vi "ATF - DD Datalog and Display.vi"() -> ()   [LabVIEW 2022 SP3]
doc: "Datalog and display software modified"
uses:
  Source Code/Control/SeCrTs-Enum.ctl
  Source Code/Globals/SeCrTS-DD globals.vi
panel:
  in  "Control PC IP Address":string="169.254.57.227"
  out "Backlog Storage":i32
  out "Backlog Pump":i32
  out "Logging Mode":string
  out "cmd":bool=TRUE
  out "Storage Connected?":bool
  in  "Pump IP Address":string="169.254.31.109"
  in  "Storage IP Address":string="169.254.219.4"
  out "Datalog Title":string
  in  "Exit":bool
  out "Log Period(Min)":dbl
  out "Logging?":bool
  out "Pumb Connected?":bool
  out "error Out":errorcluster
  # "ATF PUMP AND STORAGE"
  # "DATALOG AND DISPLAY SOFTWARE"
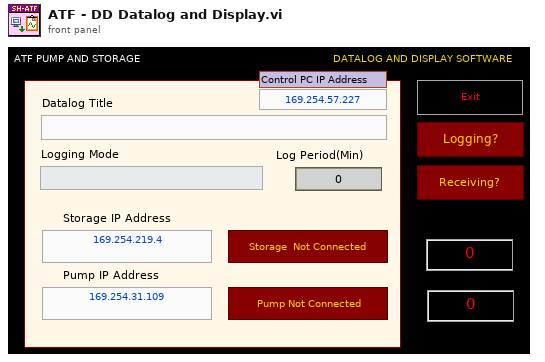
[diagram p1: front panel]
types:
  T1 = typedef "SeCrTs-Enum.ctl" = enum16{"Initialize", "Poll", "Establish ref", "Read", "Close", "Exit"}
  T2 = typedef "SeCrTS-Notifier Ref.ctl" = cluster{"Pump":refnum<notifier>, "Storage":refnum<notifier>}
  T3 = enum8{"Enabled", "Disabled", "Disabled and Grayed Out"}
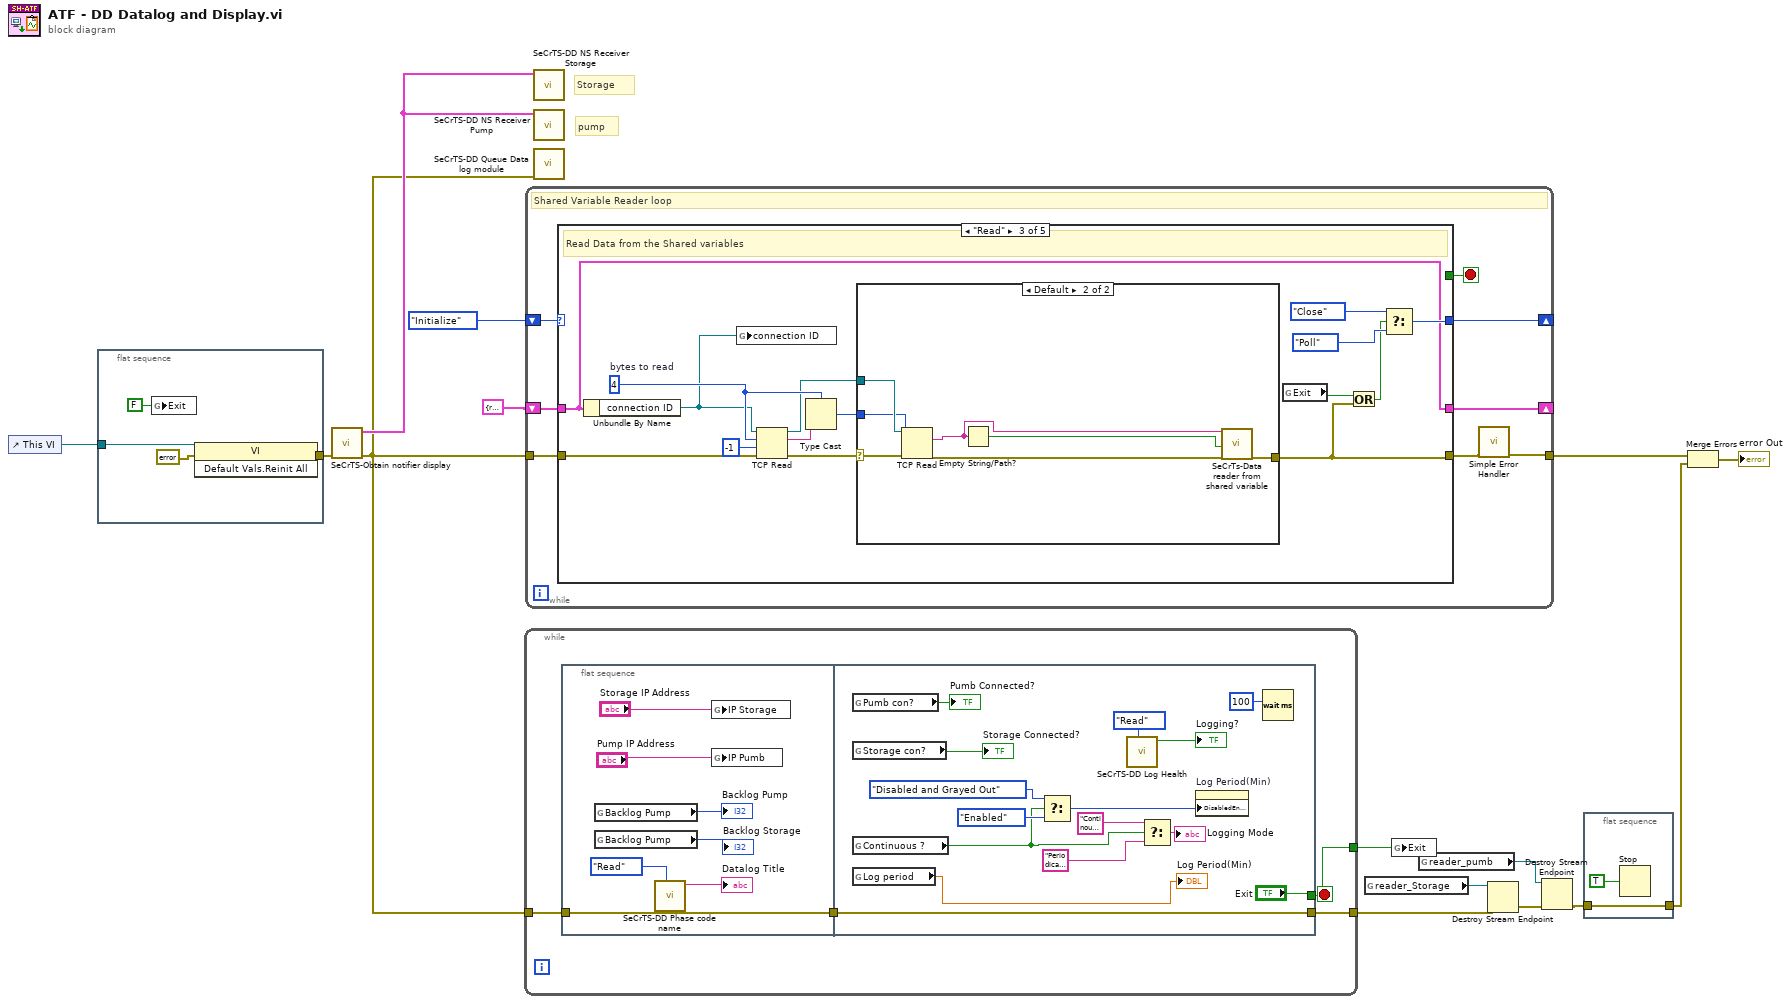
[diagram p0: block diagram]
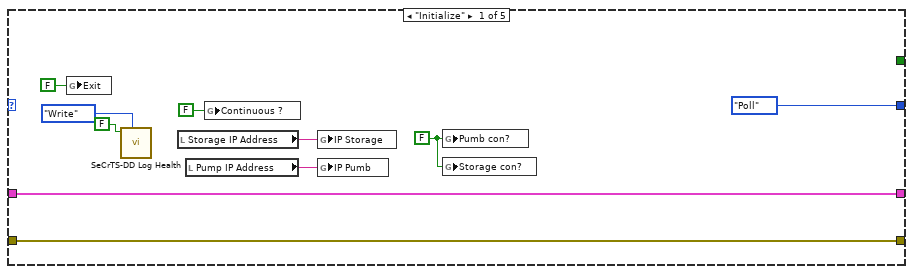
[diagram p2: hidden frame]
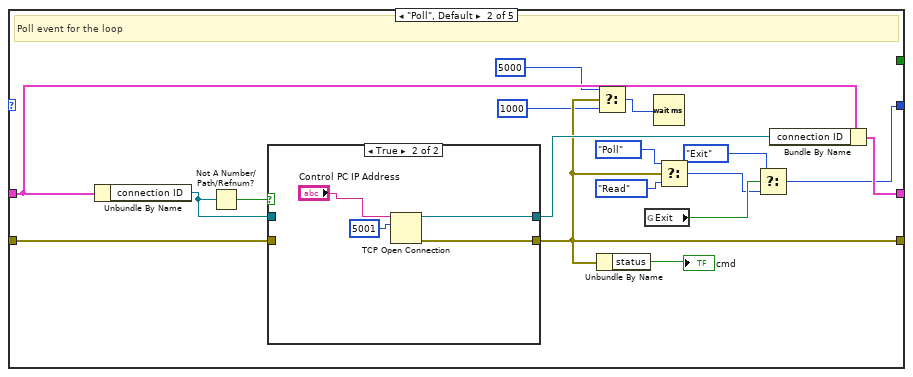
[diagram p3: hidden frame]
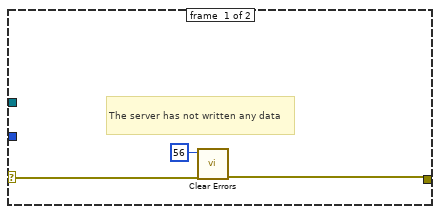
[diagram p5: hidden frame]
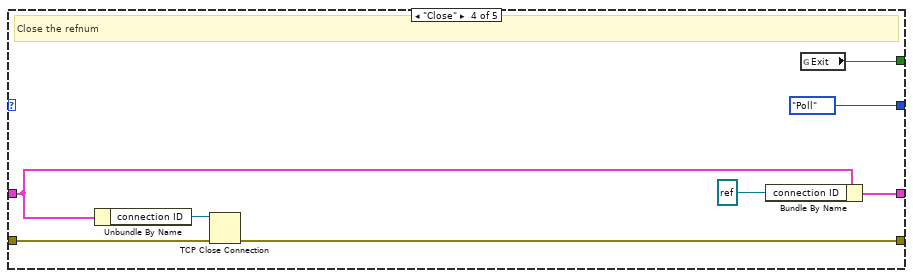
[diagram p6: hidden frame]
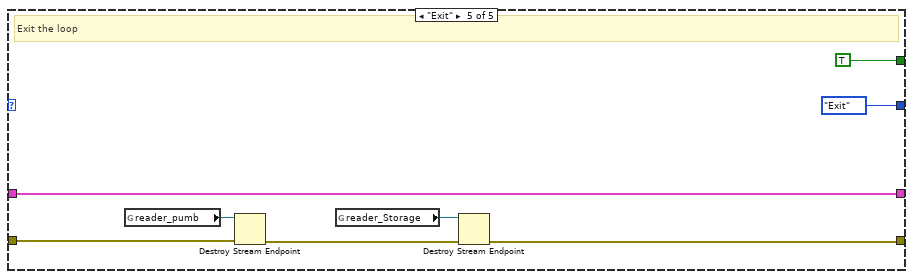
[diagram p7: hidden frame]
diagram:
  # "pump"
  # "Storage"
  n1 = control-ref of="This VI"() -> (w14:refnum<vi>)
  n2 = flat-sequence {
    tunnel: w14 -> [w19]
    tunnel: [w17] -> w11
    frame #0 {
      n3 = global write "SeCrTS-DD globals.vi" "Exit"(FALSE ("Exit")) -> ()
      n4 = invoke class="VI" method="Default Vals.Reinit All"(reference=w19, error in=errorcluster {"status"=FALSE, "code"=0, "source"=""}) -> (error out=w17:errorcluster)  [unwired: 1 in, 2 out]
    }
  }
  n5 = call "SeCrTS-Obtain notifier display.vi"("error in (no error)"=w11) -> ("error out"=w1:errorcluster, "NOT DIS Out"=w10:T2)  [unwired: 9 in]
  n6 = while {
    tunnel: w1 -> [w23]
    tunnel: [w21] -> w6
    tunnel: [w20] -> w9
    stop <- w20 stop-if-true
    n7 = flat-sequence {
      tunnel: w23 -> [w29]
      tunnel: [w29] -> w22
      tunnel: w22 -> [w38]
      tunnel: [w38] -> w21
      tunnel: ["Exit"] -> w20
      frame #0 {
        n8 = global read "SeCrTS-DD globals.vi" "Backlog Pump"() -> (→"Backlog Pump":i32)
        n9 = global read "SeCrTS-DD globals.vi" "Backlog Pump"() -> (→"Backlog Storage":i32)
        n10 = call "SeCrTS-DD Phase code name.vi"("Enum"=enum16{"Read", "Write"}."Read") -> ("Phase codeR"=→"Datalog Title":string)  [unwired: 9 in, 1 out]
        n11 = global write "SeCrTS-DD globals.vi" "IP Storage"("Storage IP Address") -> ()
        n12 = global write "SeCrTS-DD globals.vi" "IP Pumb"("Pump IP Address") -> ()
      }
      frame #1 {
        n13 = global read "SeCrTS-DD globals.vi" "Pumb con?"() -> (→"Pumb Connected?":bool)
        n14 = global read "SeCrTS-DD globals.vi" "Storage con?"() -> (→"Storage Connected?":bool)
        n15 = global read "SeCrTS-DD globals.vi" "Continuous ?"() -> (w35:bool)
        n16 = global read "SeCrTS-DD globals.vi" "Log period"() -> (→"Log Period(Min)":dbl)
        n17 = Select(t=T3."Disabled and Grayed Out" ("Disabled"), s=w35, f=T3."Enabled" ("Disabled")) -> (s? t:f=w44:T3)
        n18 = call "SeCrTS-DD Log Health.vi"("Enum"=enum16{"Read", "Write"}."Read") -> ("Log health R"=→"Logging?":bool)  [unwired: 9 in, 1 out]
        n19 = Select(t="Continous Logging Enabled" ("Logging Mode"), s=w35, f="Periodical Logging Enabled" ("Logging Mode")) -> (s? t:f=→"Logging Mode":string)
        n20 = property on="Log Period(Min)" class="DigNum (strict)"("DisabledEnum"=w44) -> ()  [unwired: 2 in, 2 out]
        n21 = Wait (ms)(milliseconds to wait=u32 100) -> ()  [unwired: 1 out]
      }
    }
  }
  n22 = while {
    shift-right: [w51] -> _
    shift-left: SeCrTs-Enum."Initialize" -> [w53]
    shift-right: [w49] -> _
    shift-left: cluster{"connection ID":refnum<k5>} {"connection ID"=refnum} -> [w50]
    tunnel: w1 -> [w52]
    tunnel: [w46] -> w12
    stop <- w48 stop-if-true
    # "Shared Variable Reader loop"
    n23 = case shown="\"Read\"" w53 {
      tunnel: w52 -> [w54 w75 w98 w117 w122]
      tunnel: [w54 w66 w89 w116 w120] -> w47
      tunnel: [SeCrTs-Enum."Poll" w69 w94 SeCrTs-Enum."Poll" SeCrTs-Enum."Exit"] -> w51
      tunnel: w50 -> [w62 w79 w93 w114 w125]
      tunnel: [w62 w80 w93 w115 w125] -> w49
      tunnel: [_ _ _ w112 TRUE] -> w48
      frame "Initialize" {
        w61 = FALSE ("Connect?")
        n24 = global write "SeCrTS-DD globals.vi" "Exit"(FALSE ("EXIT")) -> ()
        n25 = call "SeCrTS-DD Log Health.vi"("Enum"=enum16{"Read", "Write"}."Write", "Log health"=FALSE) -> ()  [unwired: 8 in, 2 out]
        n26 = local read "Storage IP Address"() -> (w60:string)
        n27 = local read "Pump IP Address"() -> (w56:string)
        n28 = global write "SeCrTS-DD globals.vi" "Continuous ?"(FALSE ("Continuous ?")) -> ()
        n29 = global write "SeCrTS-DD globals.vi" "IP Storage"(w60) -> ()
        n30 = global write "SeCrTS-DD globals.vi" "IP Pumb"(w56) -> ()
        n31 = global write "SeCrTS-DD globals.vi" "Pumb con?"(w61) -> ()
        n32 = global write "SeCrTS-DD globals.vi" "Storage con?"(w61) -> ()
      }
      frame "Poll", Default {
        # "Poll event for the loop"
        n33 = Unbundle By Name(w79) -> ("connection ID"=w77:refnum<k5>)
        n34 = Not A Number/Path/Refnum?(number/path/refnum=w77) -> (NaN/Path/Refnum?=w78:bool)
        n35 = case shown="True" w78 {
          tunnel: [w82 w84] -> w73
          tunnel: w77 -> [w82 _]
          tunnel: [w81 w86] -> w66
          tunnel: w75 -> [w81 _]
          frame False {
          }
          frame True {
            n36 = TCP Open Connection(address="Control PC IP Address", remote port or service name=u16 5001) -> (connection ID=w84:refnum<k5>, error out=w86:errorcluster)  [unwired: 3 in]
          }
        }
        n37 = Select(t=u32 5000 ("milliseconds to wait"), s=w66, f=u32 1000) -> (s? t:f=w64:u32)
        n38 = Unbundle By Name(w66) -> ("status"=→"cmd":bool)
        n39 = global read "SeCrTS-DD globals.vi" "Exit"() -> (w72:bool)
        n40 = Wait (ms)(milliseconds to wait=w64) -> ()  [unwired: 1 out]
        n41 = Select(t=SeCrTs-Enum."Poll", s=w66, f=SeCrTs-Enum."Read") -> (s? t:f=w71:T1)
        n42 = Select(t=SeCrTs-Enum."Exit", s=w72, f=w71) -> (s? t:f=w69:T1)
        n43 = Bundle By Name(cluster=w79, "connection ID"=w73) -> (w80:cluster{"connection ID":refnum<k5>})
      }
      frame "Read" {
        w100 = 4  # bytes to read
        # "Read Data from the Shared variables"
        n44 = Unbundle By Name(w93) -> ("connection ID"=w87:refnum<k5>)
        n45 = global write "SeCrTS-DD globals.vi" "connection ID"(w87) -> ()
        n46 = TCP Read(connection ID=w87, bytes to read=w100, error in (no error)=w98, 9:-1 ("timeout ms (25000)")) -> (connection ID out=w97:refnum<k5>, data out=w101:string, error out=w92:errorcluster)  [unwired: 1 in]
        n47 = Type Cast(type=w100, x=w101) -> (*(type *) &x=w99:i32)
        n48 = case shown="Default" w92 {
          selector: w92 -> [w104 w110]
          tunnel: w97 -> [_ w111]
          tunnel: [w103 w108] -> w89
          tunnel: w99 -> [_ w109]
          frame #0 {
            # "The server has not written any data"
            n49 = call <vilib>:"Clear Errors.vi"("error in (no error)"=w104, "specific error code to clear (0: all)"=56) -> ("error out"=w103:errorcluster)  [unwired: 4 in, 1 out]
          }
          frame #1 {
            n50 = TCP Read(connection ID=w111, bytes to read=w109, error in (no error)=w110) -> (data out=w105:string, error out=w107:errorcluster)  [unwired: 2 in, 1 out]
            n51 = Empty String/Path?(string/path=w105) -> (empty?=w106:bool)
            n52 = call "SeCrTs-Data reader from shared variable.vi"("Data in"=w105, "empty?"=w106, "error IO"=w107) -> ("error out"=w108:errorcluster)  [unwired: 16 in]
          }
        }
        n53 = global read "SeCrTS-DD globals.vi" "Exit"() -> (w90:bool)
        n54 = Or(x=w90, y=w89) -> (x .or. y?=w88:bool)
        n55 = Select(t=SeCrTs-Enum."Close", s=w88, f=SeCrTs-Enum."Poll") -> (s? t:f=w94:T1)
      }
      frame "Close" {
        # "Close the refnum"
        n56 = Unbundle By Name(w114) -> ("connection ID"=w118:refnum<k5>)
        n57 = TCP Close Connection(connection ID=w118, error in (no error)=w117) -> (error out=w116:errorcluster)  [unwired: 1 in, 1 out]
        n58 = Bundle By Name(cluster=w114, "connection ID"=refnum<k5> refnum) -> (w115:cluster{"connection ID":refnum<k5>})
        n59 = global read "SeCrTS-DD globals.vi" "Exit"() -> (w112:bool)
      }
      frame "Exit" {
        # "Exit the loop"
        n60 = global read "SeCrTS-DD globals.vi" "reader_pumb"() -> (w124:refnum<k21>)
        n61 = Destroy Stream Endpoint(8:w122, 11:w124) -> (0:w121:errorcluster)
        n62 = global read "SeCrTS-DD globals.vi" "reader_Storage"() -> (w123:refnum<k21>)
        n63 = Destroy Stream Endpoint(8:w121, 11:w123) -> (0:w120:errorcluster)
      }
    }
    n64 = call <vilib>:"Simple Error Handler.vi"("error in (no error)"=w47) -> ("error out"=w46:errorcluster)  [unwired: 4 in, 4 out]
  }
  n65 = call "SeCrTS-DD NS Receiver Storage.vi"("NOT DIS Out"=w10) -> ()  [unwired: 11 in]
  n66 = call "SeCrTS-DD NS Receiver Pump.vi"("NOT DIS Out"=w10) -> ()  [unwired: 11 in]
  n67 = call "SeCrTS-DD Queue Data log module.vi"("error in"=w1) -> ()  [unwired: 10 in, 1 out]
  n68 = global read "SeCrTS-DD globals.vi" "reader_Storage"() -> (w7:refnum<k21>)
  n69 = global write "SeCrTS-DD globals.vi" "Exit"(w9) -> ()
  n70 = global read "SeCrTS-DD globals.vi" "reader_pumb"() -> (w8:refnum<k21>)
  n71 = Destroy Stream Endpoint(8:w6, 11:w7) -> (0:w5:errorcluster)
  n72 = Destroy Stream Endpoint(8:w5, 11:w8) -> (0:w3:errorcluster)
  n73 = flat-sequence {
    tunnel: w3 -> [w129]
    tunnel: [w129] -> w2
    frame #0 {
      n74 = Stop(stop? (T)=TRUE) -> ()
    }
  }
  n75 = Merge Errors(w12, w2) -> (→"error Out":errorcluster)
